vi "Waveform VIG.vi"(8 "error in (no error)":errorcluster, 10 "Waveform Data (value)":string, 11 "Waveform Name (tag)":string) -> (0 "error out":errorcluster, 2 "Waveform Cluster":T1, 4 "Frozen?":bool, 5 "Live?":bool)   [LabVIEW 2017]
uses:
  controls/Waveforms.ctl
  96efe559-6eaa-4159-b87a-7768820511d5.vi
  e46816b9-7adc-4f22-a576-2816b4cd4fe7.vi
  79f1f512-6946-415a-bf1a-2fb3e1084c9b.vi
  b91dd58a-45ac-4551-9384-d6ac5957927a.vi
  b44e4c3d-e92e-4927-b867-89317095fe10.vi
  45919690-9fcc-44c5-8b4d-9a25eecad0a5.vi
  3ac2190b-ef1c-4971-b200-c90f1bcfb617.vi
  facb047e-7746-4d60-ac75-f1d13e86dbe8.vi
panel:
  out "Waveform Graph":waveform(dbl)[](graph)
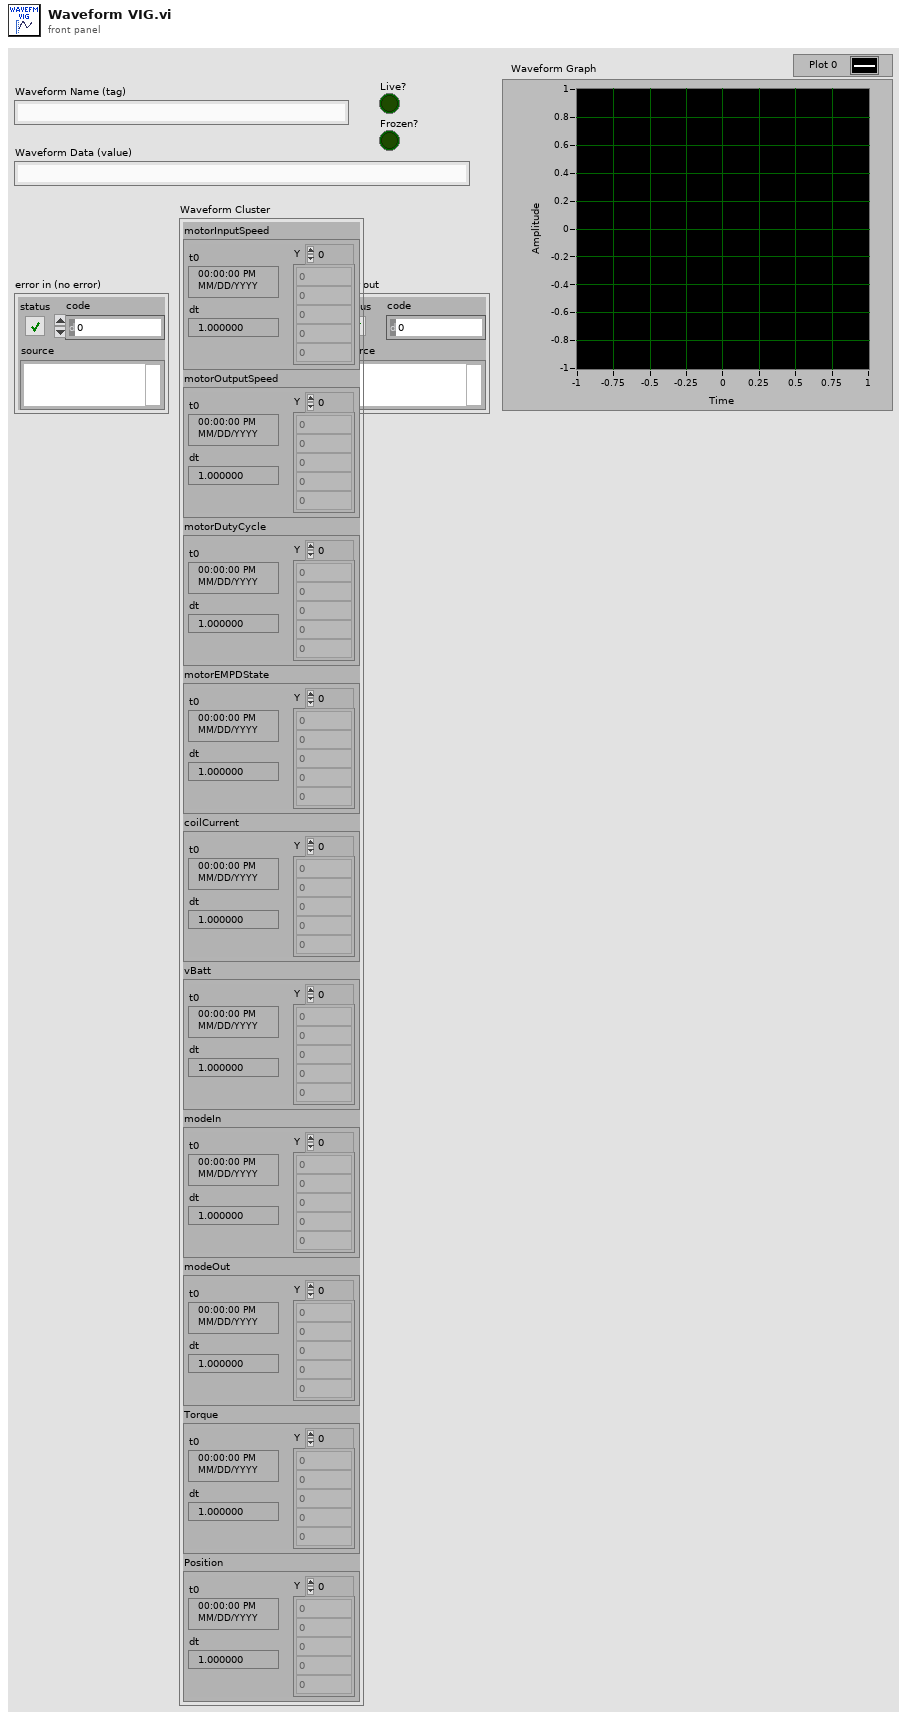
[diagram p1: front panel]
types:
  T1 = typedef "Waveforms.ctl" = cluster{"motorInputSpeed":waveform(dbl), "motorOutputSpeed":waveform(dbl), "motorDutyCycle":waveform(dbl), "motorEMPDState":waveform(dbl), "coilCurrent":waveform(dbl), "vBatt":waveform(dbl), "modeIn":waveform(dbl), "modeOut":waveform(dbl), "Torque":waveform(dbl), "Position":waveform(dbl)}
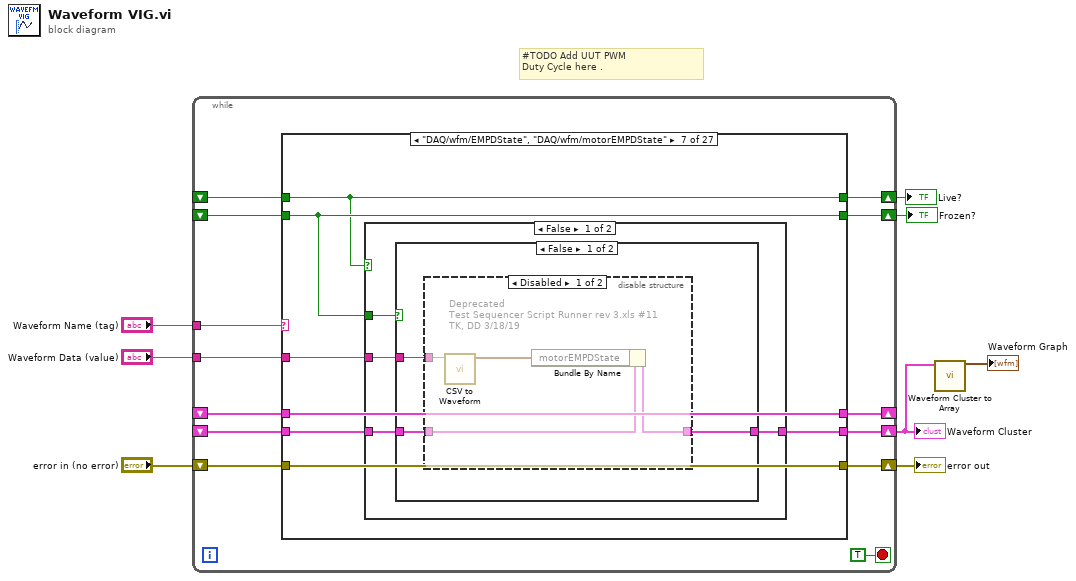
[diagram p0: block diagram]
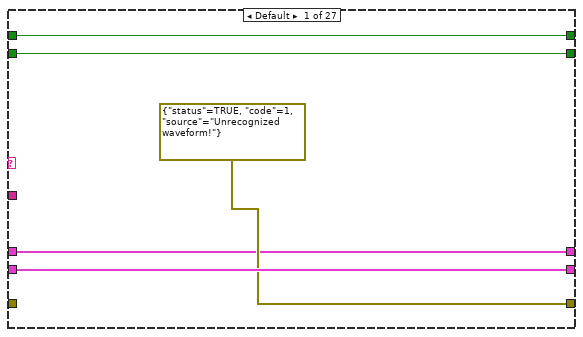
[diagram p2: hidden frame]
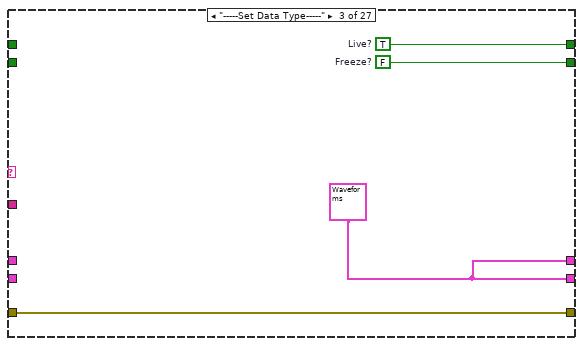
[diagram p4: hidden frame]
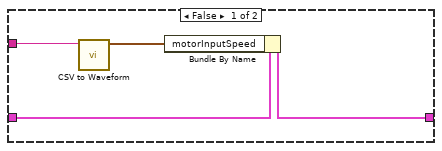
[diagram p7: hidden frame]
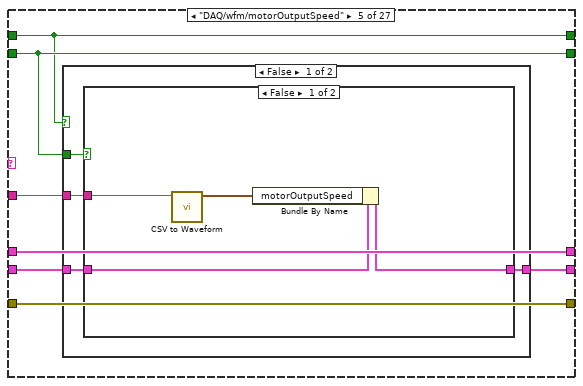
[diagram p8: hidden frame]
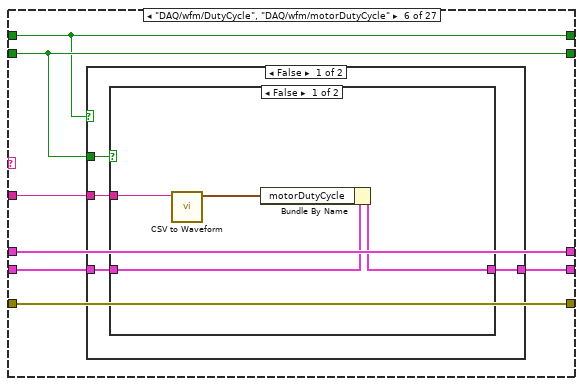
[diagram p11: hidden frame]
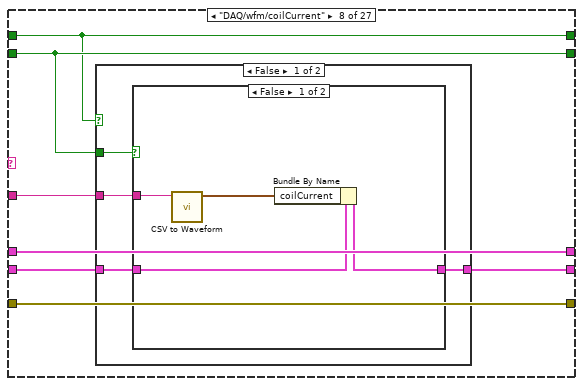
[diagram p17: hidden frame]
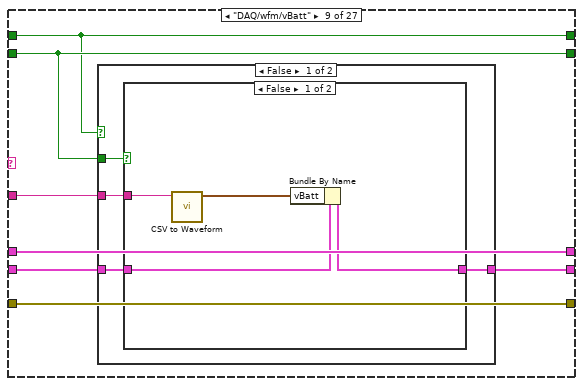
[diagram p20: hidden frame]
diagram:
  # "#TODO Add UUT PWM\nDuty Cycle here ."
  n1 = while {
    tunnel: "Waveform Data (value)" -> [w19]
    tunnel: "Waveform Name (tag)" -> [w18]
    shift-right: [w21] -> w8
    shift-left: "error in (no error)" -> [w20]
    shift-right: [w15] -> w2
    shift-left: _ -> [w17]
    shift-right: [w14] -> w4
    shift-left: _ -> [w12]
    shift-right: [w13] -> w3
    shift-left: _ -> [w11]
    shift-right: [w10] -> _
    shift-left: _ -> [w9]
    stop <- TRUE stop-if-true
    n2 = case shown="\"DAQ/wfm/EMPDState\", \"DAQ/wfm/motorEMPDState\"" w18 {
      tunnel: w19 -> [_ _ _ w42 w59 w76 w93 w114 w131 w148 w165 w182 w199 _ _ _ _ _ _ w242 w262 w282 w302 w322 w342 w362 w382]
      tunnel: w17 -> [w26 w31 _ w40 w57 w74 w91 w112 w129 w146 w163 w180 w197 w214 w219 w224 _ _ w237 w241 w261 w281 w301 w321 w341 w361 w381]
      tunnel: [w26 w31 w32 w39 w56 w73 w90 w111 w128 w145 w162 w179 w196 w214 w219 w224 w225 w229 w237 w240 w260 w280 w300 w320 w340 w360 w380] -> w15
      tunnel: w20 -> [_ w30 w35 w41 w58 w75 w92 w113 w130 w147 w164 w181 w198 w213 w218 w223 w228 w232 w236 w245 w265 w285 w305 w325 w345 w365 w385]
      tunnel: [errorcluster {"status"=TRUE, "code"=1, "source"="Unrecognized waveform!"} ("error constant") w30 w35 w41 w58 w75 w92 w113 w130 w147 w164 w181 w198 w213 w218 w223 w228 w232 w236 w243 w263 w283 w303 w323 w343 w363 w383] -> w21
      tunnel: [w24 w29 w34 w36 w53 w70 w87 w108 w125 w142 w159 w176 w193 w212 w217 w222 TRUE FALSE w235 w238 w258 w278 w298 w318 w338 w358 w378] -> w14
      tunnel: [w23 w28 w33 w37 w54 w71 w88 w109 w126 w143 w160 w177 w194 w211 TRUE FALSE w226 w230 w234 w244 w264 w284 w304 w324 w344 w364 w384] -> w13
      tunnel: w12 -> [w24 w29 _ w36 w53 w70 w87 w108 w125 w142 w159 w176 w193 w212 w217 w222 _ _ w235 w238 w258 w278 w298 w318 w338 w358 w378]
      tunnel: w11 -> [w23 w28 _ w37 w54 w71 w88 w109 w126 w143 w160 w177 w194 w211 _ _ w226 w230 w234 w244 w264 w284 w304 w324 w344 w364 w384]
      tunnel: [w22 w27 w32 w38 w55 w72 w89 w110 w127 w144 w161 w178 w195 w210 w215 w220 w225 w229 w233 w239 w259 w279 w299 w319 w339 w359 w379] -> w10
      tunnel: w9 -> [w22 w27 _ w38 w55 w72 w89 w110 w127 w144 w161 w178 w195 w210 w215 w220 w225 w229 w233 w239 w259 w279 w299 w319 w339 w359 w379]
      frame Default {
      }
      frame "" {
        # "Just pass the waveform out"
      }
      frame "-----Set Data Type-----" {
        w33 = FALSE  # Freeze?
        w34 = TRUE  # Live?
        w32 = T1 {"motorInputSpeed"={"t0"=timestamp(0 s since 1904-01-01), "dt"=1.0, "Y"=[]}, "motorOutputSpeed"={"t0"=timestamp(0 s since 1904-01-01), "dt"=1.0, "Y"=[]}, "motorDutyCycle"={"t0"=timestamp(0 s since 1904-01-01), "dt"=1.0, "Y"=[]}, "motorEMPDState"={"t0"=timestamp(0 s since 1904-01-01), "dt"=1.0, "Y"=[]}, "coilCurrent"={"t0"=timestamp(0 s since 1904-01-01), "dt"=1.0, "Y"=[]}, "vBatt"={"t0"=timestamp(0 s since 1904-01-01), "dt"=1.0, "Y"=[]}, "modeIn"={"t0"=timestamp(0 s since 1904-01-01), "dt"=1.0, "Y"=[]}, "modeOut"={"t0"=timestamp(0 s since 1904-01-01), "dt"=1.0, "Y"=[]}, "Torque"={"t0"=timestamp(0 s since 1904-01-01), "dt"=1.0, "Y"=[]}, "Position"={"t0"=timestamp(0 s since 1904-01-01), "dt"=1.0, "Y"=[]}} ("Waveform Cluster")
      }
      frame "DAQ/wfm/motorInputSpeed" {
        n3 = case shown="True" w36 {
          tunnel: w42 -> [w46 _]
          tunnel: w40 -> [w45 w52]
          tunnel: [w44 w52] -> w39
          tunnel: w37 -> [w43 _]
          frame False {
            n4 = case shown="True" w43 {
              tunnel: w46 -> [w50 _]
              tunnel: w45 -> [w48 w51]
              tunnel: [w47 w51] -> w44
              frame False {
                n5 = call "CSV to Waveform.vi"("CSV Waveform In"=w50) -> ("Waveform Out"=w49:waveform(dbl))  [unwired: 10 in]
                n6 = Bundle By Name(cluster=w48, "motorInputSpeed"=w49) -> (w47:T1)
              }
              frame True {
              }
            }
          }
          frame True {
          }
        }
      }
      frame "DAQ/wfm/motorOutputSpeed" {
        n7 = case shown="False" w53 {
          tunnel: w59 -> [w63 _]
          tunnel: w57 -> [w62 w69]
          tunnel: [w61 w69] -> w56
          tunnel: w54 -> [w60 _]
          frame False {
            n8 = case shown="False" w60 {
              tunnel: w63 -> [w67 _]
              tunnel: w62 -> [w65 w68]
              tunnel: [w64 w68] -> w61
              frame False {
                n9 = call "CSV to Waveform.vi"("CSV Waveform In"=w67) -> ("Waveform Out"=w66:waveform(dbl))  [unwired: 10 in]
                n10 = Bundle By Name(cluster=w65, "motorOutputSpeed"=w66) -> (w64:T1)
              }
              frame True {
              }
            }
          }
          frame True {
          }
        }
      }
      frame "DAQ/wfm/DutyCycle", "DAQ/wfm/motorDutyCycle" {
        n11 = case shown="False" w70 {
          tunnel: w76 -> [w80 _]
          tunnel: w74 -> [w79 w86]
          tunnel: [w78 w86] -> w73
          tunnel: w71 -> [w77 _]
          frame False {
            n12 = case shown="False" w77 {
              tunnel: w80 -> [w84 _]
              tunnel: w79 -> [w82 w85]
              tunnel: [w81 w85] -> w78
              frame False {
                n13 = call "CSV to Waveform.vi"("CSV Waveform In"=w84) -> ("Waveform Out"=w83:waveform(dbl))  [unwired: 10 in]
                n14 = Bundle By Name(cluster=w82, "motorDutyCycle"=w83) -> (w81:T1)
              }
              frame True {
              }
            }
          }
          frame True {
          }
        }
      }
      frame "DAQ/wfm/EMPDState", "DAQ/wfm/motorEMPDState" {
        n15 = case shown="False" w87 {
          tunnel: w93 -> [w97 _]
          tunnel: w91 -> [w96 w107]
          tunnel: [w95 w107] -> w90
          tunnel: w88 -> [w94 _]
          frame False {
            n16 = case shown="False" w94 {
              tunnel: w97 -> [w100 _]
              tunnel: w96 -> [w99 w106]
              tunnel: [w98 w106] -> w95
              frame False {
                n17 = disable-structure shown="Disabled" {
                  disable-tunnel: w100 -> [w104 _]
                  disable-tunnel: w99 -> [w102 w105]
                  disable-tunnel: [w101 w105] -> w98
                  frame Disabled {
                    # "Deprecated\nTest Sequencer Script Runner rev 3.xls #11\nTK, DD 3/18/19"
                    n18 = call "CSV to Waveform.vi"("CSV Waveform In"=w104) -> ("Waveform Out"=w103:waveform(dbl))  [unwired: 10 in]
                    n19 = Bundle By Name(cluster=w102, "motorEMPDState"=w103) -> (w101:T1)
                  }
                  frame Enabled {
                  }
                }
              }
              frame True {
              }
            }
          }
          frame True {
          }
        }
      }
      frame "DAQ/wfm/coilCurrent" {
        n20 = case shown="False" w108 {
          tunnel: w114 -> [w118 _]
          tunnel: w112 -> [w117 w124]
          tunnel: [w116 w124] -> w111
          tunnel: w109 -> [w115 _]
          frame False {
            n21 = case shown="False" w115 {
              tunnel: w118 -> [w122 _]
              tunnel: w117 -> [w120 w123]
              tunnel: [w119 w123] -> w116
              frame False {
                n22 = call "CSV to Waveform.vi"("CSV Waveform In"=w122) -> ("Waveform Out"=w121:waveform(dbl))  [unwired: 10 in]
                n23 = Bundle By Name(cluster=w120, "coilCurrent"=w121) -> (w119:T1)
              }
              frame True {
              }
            }
          }
          frame True {
          }
        }
      }
      frame "DAQ/wfm/vBatt" {
        n24 = case shown="False" w125 {
          tunnel: w131 -> [w135 _]
          tunnel: w129 -> [w134 w141]
          tunnel: [w133 w141] -> w128
          tunnel: w126 -> [w132 _]
          frame False {
            n25 = case shown="False" w132 {
              tunnel: w135 -> [w139 _]
              tunnel: w134 -> [w137 w140]
              tunnel: [w136 w140] -> w133
              frame False {
                n26 = call "CSV to Waveform.vi"("CSV Waveform In"=w139) -> ("Waveform Out"=w138:waveform(dbl))  [unwired: 10 in]
                n27 = Bundle By Name(cluster=w137, "vBatt"=w138) -> (w136:T1)
              }
              frame True {
              }
            }
          }
          frame True {
          }
        }
      }
      frame "DAQ/wfm/modeIn" {
        n28 = case shown="False" w142 {
          tunnel: w148 -> [w152 _]
          tunnel: w146 -> [w151 w158]
          tunnel: [w150 w158] -> w145
          tunnel: w143 -> [w149 _]
          frame False {
            n29 = case shown="False" w149 {
              tunnel: w152 -> [w156 _]
              tunnel: w151 -> [w154 w157]
              tunnel: [w153 w157] -> w150
              frame False {
                n30 = call "CSV to Waveform.vi"("CSV Waveform In"=w156) -> ("Waveform Out"=w155:waveform(dbl))  [unwired: 10 in]
                n31 = Bundle By Name(cluster=w154, "modeIn"=w155) -> (w153:T1)
              }
              frame True {
              }
            }
          }
          frame True {
          }
        }
      }
      frame "DAQ/wfm/modeOut" {
        n32 = case shown="False" w159 {
          tunnel: w165 -> [w169 _]
          tunnel: w163 -> [w168 w175]
          tunnel: [w167 w175] -> w162
          tunnel: w160 -> [w166 _]
          frame False {
            n33 = case shown="False" w166 {
              tunnel: w169 -> [w173 _]
              tunnel: w168 -> [w171 w174]
              tunnel: [w170 w174] -> w167
              frame False {
                n34 = call "CSV to Waveform.vi"("CSV Waveform In"=w173) -> ("Waveform Out"=w172:waveform(dbl))  [unwired: 10 in]
                n35 = Bundle By Name(cluster=w171, "modeOut"=w172) -> (w170:T1)
              }
              frame True {
              }
            }
          }
          frame True {
          }
        }
      }
      frame "DAQ/wfm/torque" {
        n36 = case shown="False" w176 {
          tunnel: w182 -> [w186 _]
          tunnel: w180 -> [w185 w192]
          tunnel: [w184 w192] -> w179
          tunnel: w177 -> [w183 _]
          frame False {
            n37 = case shown="False" w183 {
              tunnel: w186 -> [w190 _]
              tunnel: w185 -> [w188 w191]
              tunnel: [w187 w191] -> w184
              frame False {
                n38 = call "CSV to Waveform.vi"("CSV Waveform In"=w190) -> ("Waveform Out"=w189:waveform(dbl))  [unwired: 10 in]
                n39 = Bundle By Name(cluster=w188, "Torque"=w189) -> (w187:T1)
              }
              frame True {
              }
            }
          }
          frame True {
          }
        }
      }
      frame "DAQ/wfm/position" {
        n40 = case shown="False" w193 {
          tunnel: w199 -> [w203 _]
          tunnel: w197 -> [w202 w209]
          tunnel: [w201 w209] -> w196
          tunnel: w194 -> [w200 _]
          frame False {
            n41 = case shown="False" w200 {
              tunnel: w203 -> [w207 _]
              tunnel: w202 -> [w205 w208]
              tunnel: [w204 w208] -> w201
              frame False {
                n42 = call "CSV to Waveform.vi"("CSV Waveform In"=w207) -> ("Waveform Out"=w206:waveform(dbl))  [unwired: 10 in]
                n43 = Bundle By Name(cluster=w205, "Position"=w206) -> (w204:T1)
              }
              frame True {
              }
            }
          }
          frame True {
          }
        }
      }
      frame "------- Config Commands -----" {
      }
      frame "Freeze" {
      }
      frame "Unfreeze" {
      }
      frame "Live" {
      }
      frame "Shift" {
      }
      frame "----- Live Data -----" {
      }
      frame "DAQ/live/FADM" {
        n44 = case shown="True" w238 {
          tunnel: w245 -> [w246 w257]
          tunnel: [w246 w256] -> w243
          tunnel: w242 -> [_ w254]
          tunnel: w241 -> [w247 w252]
          tunnel: [w247 w251] -> w240
          frame False {
          }
          frame True {
            n45 = Scan From String(input string=w254, error in=w257) -> (error out=w256:errorcluster, output 1=w248:dbl)  [unwired: 3 in, 2 out]
            n46 = Unbundle By Name(w252) -> ("modeOut"=w255:waveform(dbl))
            n47 = Unbundle By Name(w255) -> ("Y"=w249:dbl[])
            n48 = call "Limit Array Size.vim"("Numeric"=w248, "Array in"=w249) -> ("Array out"=w250:dbl[])  [unwired: 5 in]
            n49 = Bundle By Name(cluster=w255, "Y"=w250) -> (w253:waveform(dbl))
            n50 = Bundle By Name(cluster=w252, "modeOut"=w253) -> (w251:T1)
          }
        }
      }
      frame "DAQ/live/FADR" {
        n51 = case shown="True" w258 {
          tunnel: w265 -> [w266 w277]
          tunnel: [w266 w276] -> w263
          tunnel: w262 -> [_ w274]
          tunnel: w261 -> [w267 w272]
          tunnel: [w267 w271] -> w260
          frame False {
          }
          frame True {
            n52 = Scan From String(input string=w274, error in=w277) -> (error out=w276:errorcluster, output 1=w268:dbl)  [unwired: 3 in, 2 out]
            n53 = Unbundle By Name(w272) -> ("modeIn"=w275:waveform(dbl))
            n54 = Unbundle By Name(w275) -> ("Y"=w269:dbl[])
            n55 = call "Limit Array Size.vim"("Numeric"=w268, "Array in"=w269) -> ("Array out"=w270:dbl[])  [unwired: 5 in]
            n56 = Bundle By Name(cluster=w275, "Y"=w270) -> (w273:waveform(dbl))
            n57 = Bundle By Name(cluster=w272, "modeIn"=w273) -> (w271:T1)
          }
        }
      }
      frame "DAQ/live/coilCurrent" {
        n58 = case shown="True" w278 {
          tunnel: w285 -> [w286 w297]
          tunnel: [w286 w296] -> w283
          tunnel: w282 -> [_ w294]
          tunnel: w281 -> [w287 w292]
          tunnel: [w287 w291] -> w280
          frame False {
          }
          frame True {
            n59 = Scan From String(input string=w294, error in=w297) -> (error out=w296:errorcluster, output 1=w288:dbl)  [unwired: 3 in, 2 out]
            n60 = Unbundle By Name(w292) -> ("coilCurrent"=w295:waveform(dbl))
            n61 = Unbundle By Name(w295) -> ("Y"=w289:dbl[])
            n62 = call "Limit Array Size.vim"("Numeric"=w288, "Array in"=w289) -> ("Array out"=w290:dbl[])  [unwired: 5 in]
            n63 = Bundle By Name(cluster=w295, "Y"=w290) -> (w293:waveform(dbl))
            n64 = Bundle By Name(cluster=w292, "coilCurrent"=w293) -> (w291:T1)
          }
        }
      }
      frame "DAQ/live/position" {
        n65 = case shown="True" w298 {
          tunnel: w305 -> [w306 w317]
          tunnel: [w306 w316] -> w303
          tunnel: w302 -> [_ w314]
          tunnel: w301 -> [w307 w312]
          tunnel: [w307 w311] -> w300
          frame False {
          }
          frame True {
            n66 = Scan From String(input string=w314, error in=w317) -> (error out=w316:errorcluster, output 1=w308:dbl)  [unwired: 3 in, 2 out]
            n67 = Unbundle By Name(w312) -> ("Position"=w315:waveform(dbl))
            n68 = Unbundle By Name(w315) -> ("Y"=w309:dbl[])
            n69 = call "Limit Array Size.vim"("Numeric"=w308, "Array in"=w309) -> ("Array out"=w310:dbl[])  [unwired: 5 in]
            n70 = Bundle By Name(cluster=w315, "Y"=w310) -> (w313:waveform(dbl))
            n71 = Bundle By Name(cluster=w312, "Position"=w313) -> (w311:T1)
          }
        }
      }
      frame "DAQ/live/inputSpeed" {
        n72 = case shown="True" w318 {
          tunnel: w325 -> [w326 w337]
          tunnel: [w326 w336] -> w323
          tunnel: w322 -> [_ w334]
          tunnel: w321 -> [w327 w332]
          tunnel: [w327 w331] -> w320
          frame False {
          }
          frame True {
            n73 = Unbundle By Name(w332) -> ("motorInputSpeed"=w335:waveform(dbl))
            n74 = Scan From String(input string=w334, error in=w337) -> (error out=w336:errorcluster, output 1=w328:dbl)  [unwired: 3 in, 2 out]
            n75 = Unbundle By Name(w335) -> ("Y"=w329:dbl[])
            n76 = call "Limit Array Size.vim"("Numeric"=w328, "Array in"=w329) -> ("Array out"=w330:dbl[])  [unwired: 5 in]
            n77 = Bundle By Name(cluster=w335, "Y"=w330) -> (w333:waveform(dbl))
            n78 = Bundle By Name(cluster=w332, "motorInputSpeed"=w333) -> (w331:T1)
          }
        }
      }
      frame "DAQ/live/outputSpeed" {
        n79 = case shown="True" w338 {
          tunnel: w345 -> [w346 w357]
          tunnel: [w346 w356] -> w343
          tunnel: w342 -> [_ w354]
          tunnel: w341 -> [w347 w352]
          tunnel: [w347 w351] -> w340
          frame False {
          }
          frame True {
            n80 = Unbundle By Name(w352) -> ("motorOutputSpeed"=w355:waveform(dbl))
            n81 = Scan From String(input string=w354, error in=w357) -> (error out=w356:errorcluster, output 1=w348:dbl)  [unwired: 3 in, 2 out]
            n82 = Unbundle By Name(w355) -> ("Y"=w349:dbl[])
            n83 = call "Limit Array Size.vim"("Numeric"=w348, "Array in"=w349) -> ("Array out"=w350:dbl[])  [unwired: 5 in]
            n84 = Bundle By Name(cluster=w355, "Y"=w350) -> (w353:waveform(dbl))
            n85 = Bundle By Name(cluster=w352, "motorOutputSpeed"=w353) -> (w351:T1)
          }
        }
      }
      frame "DAQ/live/torque" {
        n86 = case shown="True" w358 {
          tunnel: w365 -> [w366 w377]
          tunnel: [w366 w376] -> w363
          tunnel: w362 -> [_ w374]
          tunnel: w361 -> [w367 w372]
          tunnel: [w367 w371] -> w360
          frame False {
          }
          frame True {
            n87 = Scan From String(input string=w374, error in=w377) -> (error out=w376:errorcluster, output 1=w368:dbl)  [unwired: 3 in, 2 out]
            n88 = Unbundle By Name(w372) -> ("Torque"=w375:waveform(dbl))
            n89 = Unbundle By Name(w375) -> ("Y"=w369:dbl[])
            n90 = call "Limit Array Size.vim"("Numeric"=w368, "Array in"=w369) -> ("Array out"=w370:dbl[])  [unwired: 5 in]
            n91 = Bundle By Name(cluster=w375, "Y"=w370) -> (w373:waveform(dbl))
            n92 = Bundle By Name(cluster=w372, "Torque"=w373) -> (w371:T1)
          }
        }
      }
      frame "DAQ/live/vbatt" {
        n93 = case shown="True" w378 {
          tunnel: w385 -> [w386 w397]
          tunnel: [w386 w396] -> w383
          tunnel: w382 -> [_ w394]
          tunnel: w381 -> [w387 w392]
          tunnel: [w387 w391] -> w380
          frame False {
          }
          frame True {
            n94 = Scan From String(input string=w394, error in=w397) -> (error out=w396:errorcluster, output 1=w388:dbl)  [unwired: 3 in, 2 out]
            n95 = Unbundle By Name(w392) -> ("vBatt"=w395:waveform(dbl))
            n96 = Unbundle By Name(w395) -> ("Y"=w389:dbl[])
            n97 = call "Limit Array Size.vim"("Numeric"=w388, "Array in"=w389) -> ("Array out"=w390:dbl[])  [unwired: 5 in]
            n98 = Bundle By Name(cluster=w395, "Y"=w390) -> (w393:waveform(dbl))
            n99 = Bundle By Name(cluster=w392, "vBatt"=w393) -> (w391:T1)
          }
        }
      }
    }
  }
  "error out" <- w8
  "Waveform Cluster" <- w2
  "Live?" <- w4
  "Frozen?" <- w3
  n100 = call "Waveform Cluster to Array.vi"("Waveform Cluster"=w2) -> ("Array"=→"Waveform Graph":waveform(dbl)[])  [unwired: 10 in]
